vi "Prueba_HTTP_V0.2.vi"() -> ()   [LabVIEW 2011]
uses:
  mbed/Transport Mechanisms/HTTPRPC/HTTPRPC.lvclass
panel:
  in  "Dirección IP":string="192.168.1.2"
  in  "stop":bool
  in  "Vout":dbl(slide) scale=-10.0..10.0
  in  "Direccion":bool
  in  "Frecuencia":u32(slide) scale=0.0..30000.0
  # "PRUEBA Comunicacion HTTP v0.1 - Deslizador"
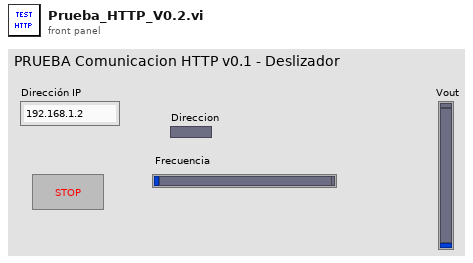
[diagram p1: front panel]
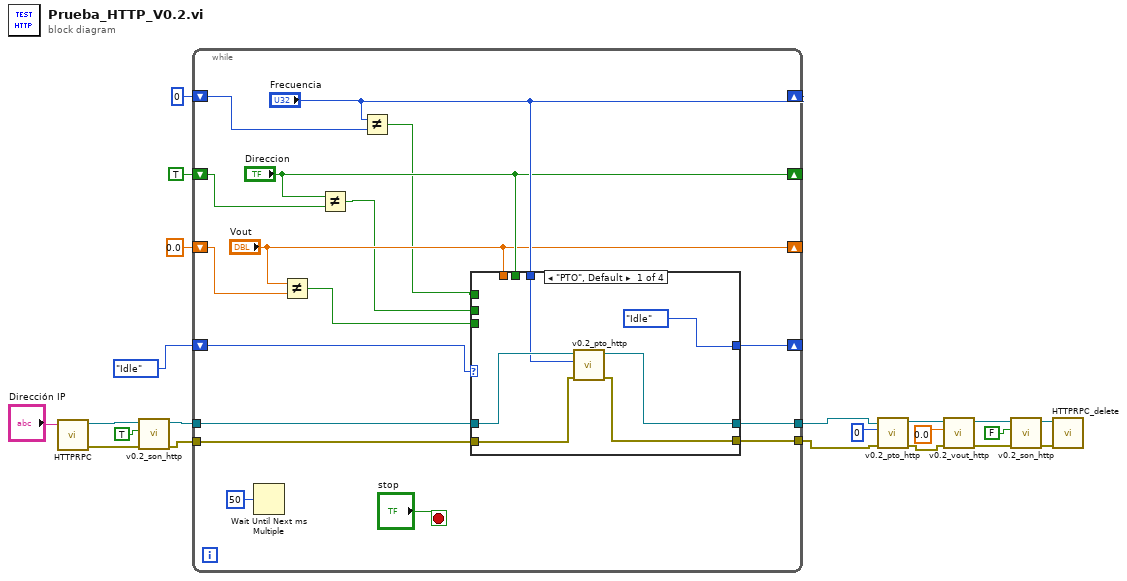
[diagram p0: block diagram]
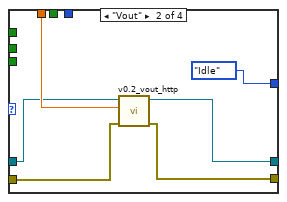
[diagram p2: hidden frame]
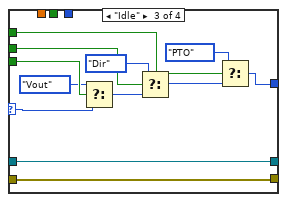
[diagram p3: hidden frame]
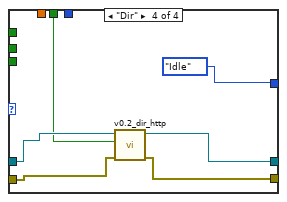
[diagram p4: hidden frame]
diagram:
  n1 = call "HTTPRPC.vi"("Address"="Dirección IP") -> ("error out"=w6:errorcluster, "mbed.lvclass"=w21:refnum<class "mbed.lvclass">)  [unwired: 7 in]
  n2 = call "v0.2_son_http.vi"("error in"=w6, "ServoON"=TRUE, "mbed.lvclass IN"=w21) -> ("error out"=w5:errorcluster, "mbed.lvclass OUT"=w20:refnum<class "mbed.lvclass">)  [unwired: 7 in]
  n3 = while {
    tunnel: [w32] -> w14
    tunnel: w20 -> [w31]
    shift-right: ["Frecuencia"] -> _
    shift-left: u32 0 ("Frecuencia") -> [w36]
    shift-right: ["Direccion"] -> _
    shift-left: TRUE ("Direccion") -> [w35]
    shift-right: ["Vout"] -> _
    shift-left: 0.0 ("Vout") -> [w34]
    shift-right: [w30] -> _
    shift-left: enum16{"Idle", "PTO", "Vout", "Dir"}."Idle" -> [w33]
    tunnel: w5 -> [w25]
    tunnel: [w24] -> w4
    stop <- "stop" stop-if-true
    n4 = Wait Until Next ms Multiple(millisecond multiple=u32 50) -> ()  [unwired: 1 out]
    n5 = Not Equal?(x="Vout", y=w34) -> (x != y?=w29:bool)
    n6 = Not Equal?(x="Direccion", y=w35) -> (x != y?=w22:bool)
    n7 = Not Equal?(x="Frecuencia", y=w36) -> (x != y?=w23:bool)
    n8 = case shown="\"PTO\", Default" w33 {
      selector: w33 -> [_ _ w60 _]
      tunnel: [w43 w48 w62 w65] -> w32
      tunnel: w31 -> [w44 w49 w62 w68]
      tunnel: [enum16{"Idle", "PTO", "Vout", "Dir"}."Idle" enum16{"Idle", "PTO", "Vout", "Dir"}."Idle" w61 enum16{"Idle", "PTO", "Vout", "Dir"}."Idle"] -> w30
      tunnel: w23 -> [_ _ w59 _]
      tunnel: w29 -> [_ _ w58 _]
      tunnel: "Frecuencia" -> [w42 _ _ _]
      tunnel: "Direccion" -> [_ _ _ w66]
      tunnel: "Vout" -> [_ w50 _ _]
      tunnel: w25 -> [w41 w47 w57 w67]
      tunnel: [w40 w46 w57 w64] -> w24
      tunnel: w22 -> [_ _ w53 _]
      frame "PTO", Default {
        n9 = call "v0.2_pto_http.vi"("error in"=w41, "Frecuencia"=w42, "mbed.lvclass IN"=w44) -> ("error out"=w40:errorcluster, "mbed.lvclass OUT"=w43:refnum<class "mbed.lvclass">)  [unwired: 7 in]
      }
      frame "Vout" {
        n10 = call "v0.2_vout_http.vi"("error in (no error)"=w47, "Vout"=w50, "mbed.lvclass IN"=w49) -> ("error out"=w46:errorcluster, "mbed.lvclass OUT"=w48:refnum<class "mbed.lvclass">)  [unwired: 7 in]
      }
      frame "Idle" {
        n11 = Select(t=enum16{"Idle", "PTO", "Vout", "Dir"}."Vout", s=w58, f=w60) -> (s? t:f=w52:enum16{"Idle", "PTO", "Vout", "Dir"})
        n12 = Select(t=enum16{"Idle", "PTO", "Vout", "Dir"}."Dir", s=w53, f=w52) -> (s? t:f=w51:enum16{"Idle", "PTO", "Vout", "Dir"})
        n13 = Select(t=enum16{"Idle", "PTO", "Vout", "Dir"}."PTO", s=w59, f=w51) -> (s? t:f=w61:enum16{"Idle", "PTO", "Vout", "Dir"})
      }
      frame "Dir" {
        n14 = call "v0.2_dir_http.vi"("error in (no error)"=w67, "Direccion"=w66, "mbed.lvclass IN"=w68) -> ("error out"=w64:errorcluster, "mbed.lvclass OUT"=w65:refnum<class "mbed.lvclass">)  [unwired: 7 in]
      }
    }
  }
  n15 = call "v0.2_pto_http.vi"("error in"=w4, "Frecuencia"=u32 0, "mbed.lvclass IN"=w14) -> ("error out"=w3:errorcluster, "mbed.lvclass OUT"=w13:refnum<class "mbed.lvclass">)  [unwired: 7 in]
  n16 = call "v0.2_vout_http.vi"("error in (no error)"=w3, "Vout"=0.0, "mbed.lvclass IN"=w13) -> ("error out"=w2:errorcluster, "mbed.lvclass OUT"=w12:refnum<class "mbed.lvclass">)  [unwired: 7 in]
  n17 = call "v0.2_son_http.vi"("error in"=w2, "ServoON"=FALSE, "mbed.lvclass IN"=w12) -> ("error out"=w1:errorcluster, "mbed.lvclass OUT"=w19:refnum<class "mbed.lvclass">)  [unwired: 7 in]
  n18 = call "HTTPRPC_delete.vi"("mbed_LVLibrary.lvlib:mbed.lvclass"=w19, "error in (no error)"=w1) -> ()  [unwired: 8 in, 1 out]
